vi "Cleanup Path Group.vi"(0 "Path Group in":refnum<class "Path Group.lvclass">, 5 "Path Callbacks Reference":refnum<vi>[](array[refnum]), 11 "error in":errorcluster) -> (4 "Path Group out":refnum<class "Path Group.lvclass">, 15 "error out":errorcluster)   [LabVIEW 2023, in "RFCalAndFixtureCharact.Common.lvlib"]
uses:
  RFCalAndFixtureCharact.Common.lvlib
  Base Classes/Path/Path.lvclass
  Base Classes/Path Group/Path Group.lvclass
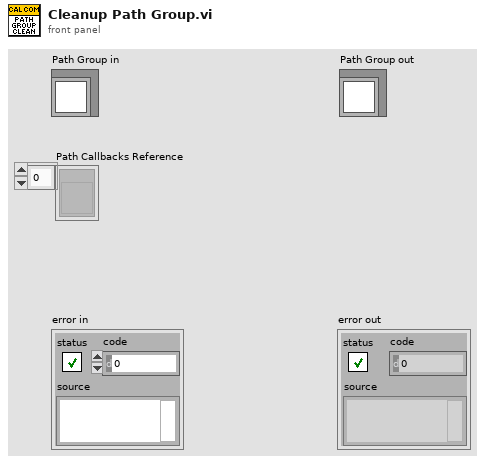
[diagram p1: front panel]
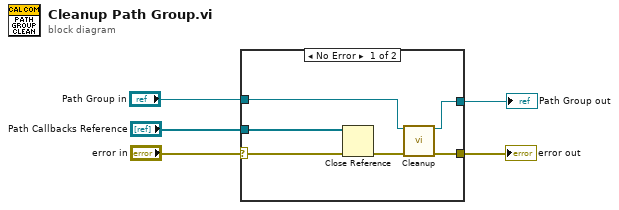
[diagram p0: block diagram]
diagram:
  n1 = case shown="No Error" "error in" {
    selector: "error in" -> [w10 w13]
    tunnel: [w8 w13] -> w4
    tunnel: "Path Callbacks Reference" -> [w11 _]
    tunnel: "Path Group in" -> [w7 w12]
    tunnel: [w6 w12] -> w1
    frame No Error {
      n2 = Close Reference(reference=w11, error in (no error)=w10) -> (error out=w9:errorcluster)
      n3 = call-dynamic "Cleanup.vi"("Path Group in"=w7, "error in (no error)"=w9) -> ("Path Group out"=w6:refnum<class "Path Group.lvclass">, "error out"=w8:errorcluster)  [unwired: 12 in]
    }
    frame Error {
    }
  }
  "error out" <- w4
  "Path Group out" <- w1
